vi "Test Lock-in amplifier API.vi"() -> ()   [LabVIEW 2020]
doc: "Lock-in amplifier API Tester."
uses:
  Lock-in amplifier.lvlib
  <vilib>/Utility/error.llb/DialogType.ctl
  Support/Filter config -- cluster.ctl
  Support/Input signal config -- typedef.ctl
  Support/Sense-Reserve config -- cluster.ctl
panel:
  in  "Sens/Reserve":T1={"Dynamic Reserve "=1, "Sensitivity"=20} {"Dynamic Reserve" items=["Auto Reserve"=-1, "High Reserve"=0, "Normal"=1, "Low Noise"=2]; "Sensitivity" items=["Auto Gain"=-1, "2 nV/fA"=0, "5 nV/fA"=1, "10 nV/fA"=2, "20 nV/fA"=3, "50 nV/fA"=4, "100 nV/fA"=5, "200 nV/fA"=6, "500 nV/fA"=7, "1 uV/pA"=8, "2 uV/pA"=9, "5 uV/pA"=10, "10 uV/pA"=11, "20 uV/pA"=12, "50 uV/pA"=13, "100 uV/pA"=14, "200 uV/pA"=15, "500 uV/pA"=16, "1 mV/nA"=17, "2 mV/nA"=18, "5 mV/nA"=19, "10 mV/nA"=20, "20 mV/nA"=21, "50 mV/nA"=22, "100 mV/nA"=23, "200 mV/nA"=24, "500 mV/mA"=25, "1 V/uA"=26]}
  in  "Input signal":T2={"Input Shield Grounding"=1, "Input Connection"=0, "Input Coupling"=1} {"Input Shield Grounding" items=["Float", "Ground"]; "Input Connection" items=["Single-Ended Voltage", "Differential Voltage", "1 MOhm Current Gain", "100 MOhm Current Gain"]; "Input Coupling" items=["AC", "DC"]}
  in  "Filter":T3={"Time Constant"=9, "Enable Sync Filter?"=FALSE, "Low Pass Filter Slope"=1} {"Low Pass Filter Slope" items=["6 dB/oct", "12 dB/oct", "18 db/oct", "24 dB/oct"]; "Time Constant" items=["10 us", "30 us", "100 us", "300 us", "1 ms", "3 ms", "10 ms", "30 ms", "100 ms", "300 ms", "1 s", "3 s", "10 s", "30 s", "100 s", "300 s", "1 ks", "3 ks", "10 ks", "30 ks"]}
  in  "Timeout":i32=100
  in  "Stop continuous acquisition":bool
  in  "Average?":bool
  in  "Start continuous acquisition":bool
  in  "Configure":bool
  out "Connected":bool
  in  "Simulate?":bool
  in  "Disconnect":bool
  in  "N samples":i32
  in  "Average samples":bool
  in  "Parameter":u16(ring)=1 items=["X"=1, "Y"=2, "R"=3, "Theta"=4, "Channel 1"=5, "Channel 2"=6, "Aux In 1"=7, "Aux In 2"=8, "Aux In 3"=9, "Aux In 4"=10]
  out "Data":dbl
  in  "Read datapoint":bool
  in  "VISA resource name":refnum<visa-resource-name>
  in  "Connect":bool
  in  "Remove Panel from Subpanel":bool
  in  "Draw Panel into Subpanel":bool
  in  "Show Diagram on Init":bool
  in  "Run as Singleton?":bool
  in  "Show Block Diagram":bool
  in  "Refresh Modules":bool
  out "Active Modules":string[](array[string])
  in  "Stop Module":bool
  in  "Select Module":i32(ring)=-1 caption="Select Module\nTo send Request to" items=["All"=-1]
  in  "Run New Module":bool
  in  "Hide Module Panel":bool
  in  "Show Module Panel":bool
  out "Status":string
  # "This VI tests the API for the Module."
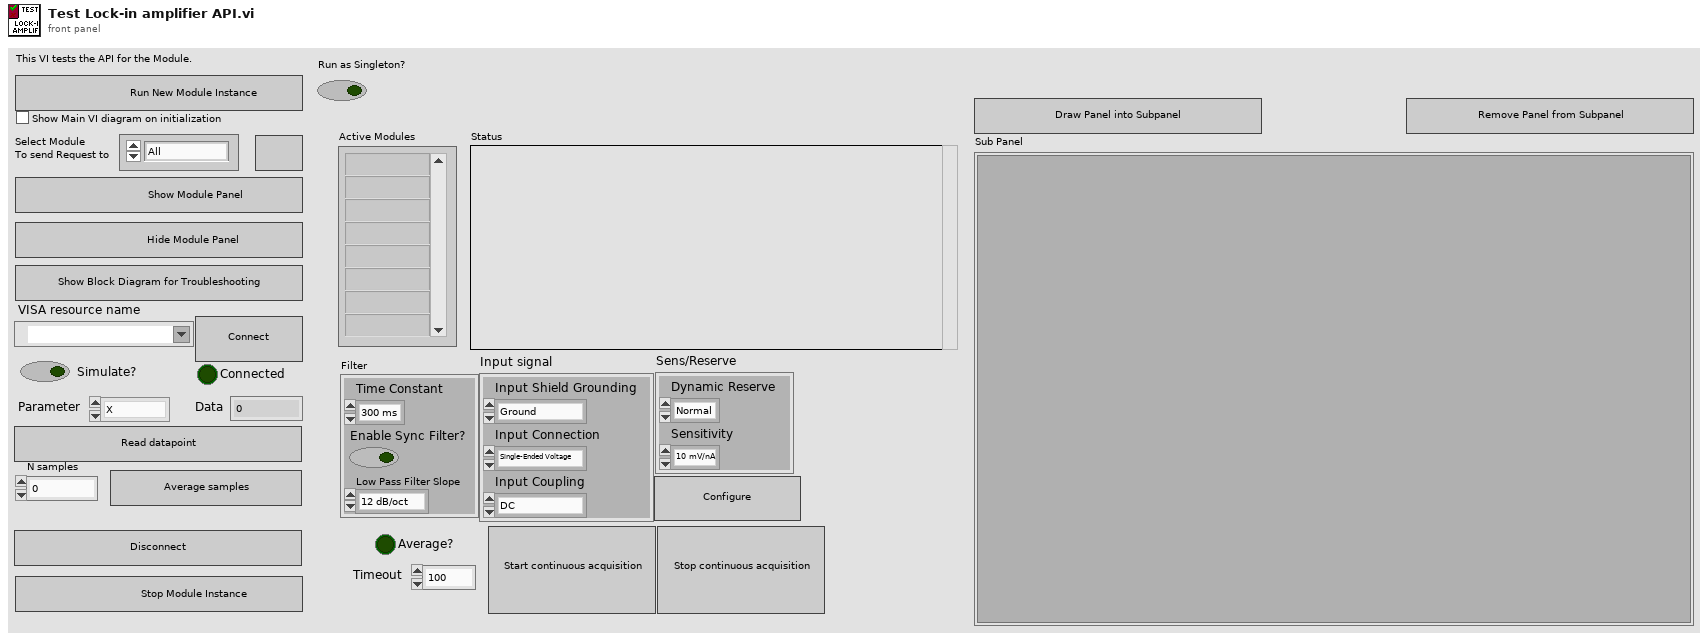
[diagram p1: front panel]
types:
  T1 = typedef "Lock-in amplifier.lvlib/Sense-Reserve config -- cluster.ctl" = cluster{"Dynamic Reserve ":i16, "Sensitivity":i16}
  T2 = typedef "Lock-in amplifier.lvlib/Input signal config -- typedef.ctl" = cluster{"Input Shield Grounding":u16, "Input Connection":u16, "Input Coupling":u16}
  T3 = typedef "Lock-in amplifier.lvlib/Filter config -- cluster.ctl" = cluster{"Time Constant":u16, "Enable Sync Filter?":bool, "Low Pass Filter Slope":u16}
  T4 = typedef "Lock-in amplifier.lvlib/Broadcast Events--cluster.ctl" = cluster{"Module Did Init":refnum<user-event>, "Status Updated":refnum<user-event>, "Error Reported":refnum<user-event>, "Module Did Stop":refnum<user-event>, "Update Module Execution Status":refnum<user-event>, "Helper Loop Status Updated":refnum<user-event>, "Data available":refnum<user-event>}
  T5 = typedef "DialogType.ctl" = u16
  T6 = typedef "Lock-in amplifier.lvlib/Helper Loop Status--enum.ctl" = enum16{"Awake", "Asleep"}
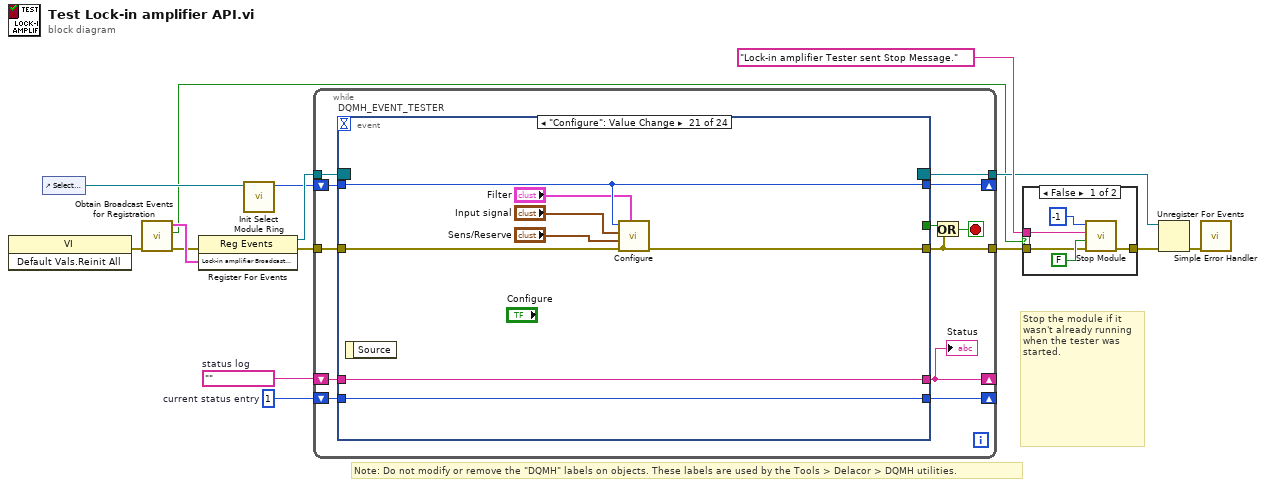
[diagram p0: block diagram]
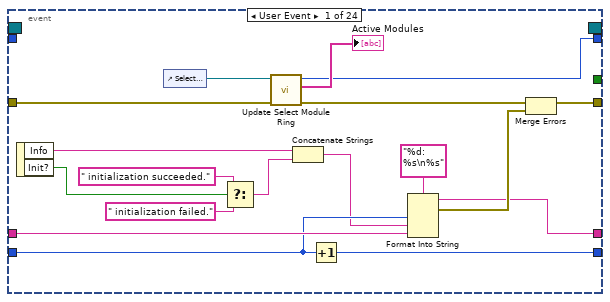
[diagram p3: hidden frame]
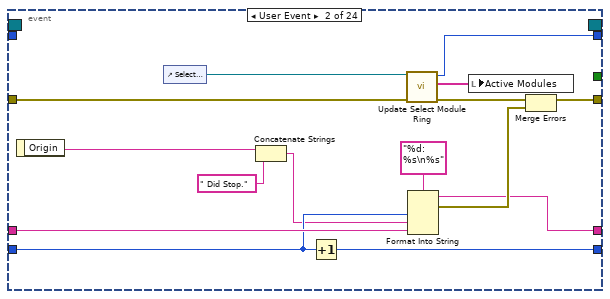
[diagram p4: hidden frame]
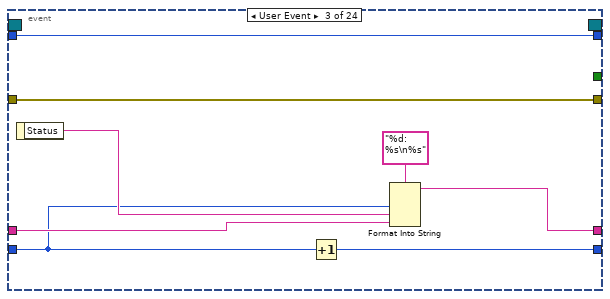
[diagram p5: hidden frame]
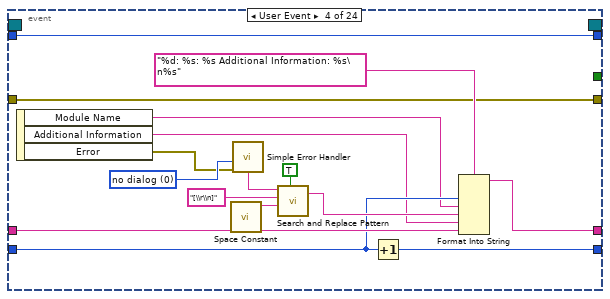
[diagram p6: hidden frame]
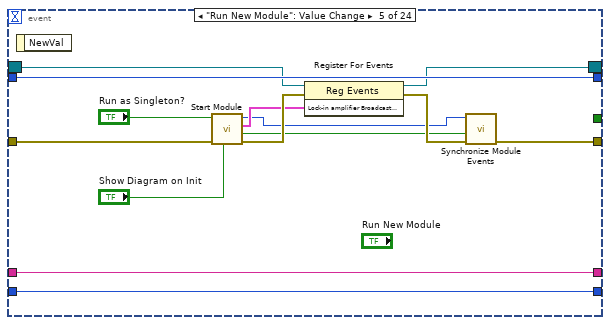
[diagram p7: hidden frame]
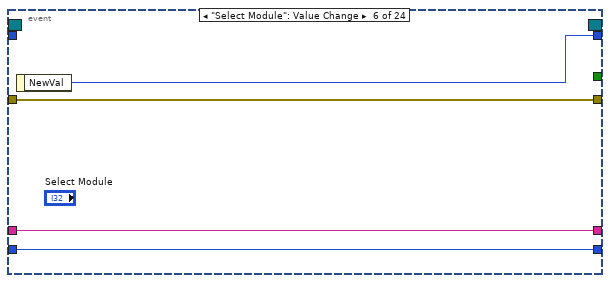
[diagram p8: hidden frame]
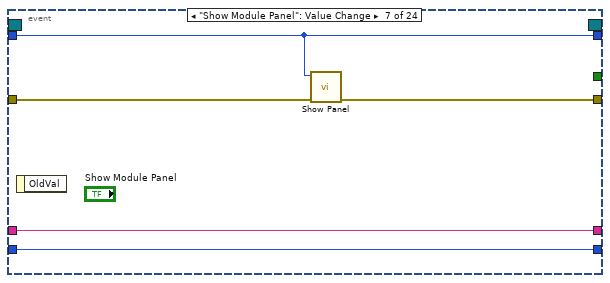
[diagram p9: hidden frame]
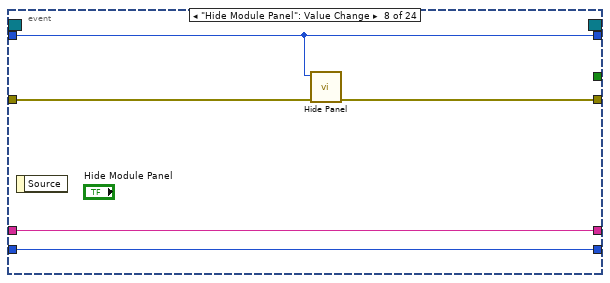
[diagram p10: hidden frame]
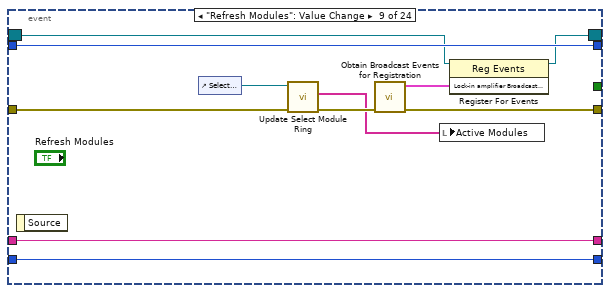
[diagram p11: hidden frame]
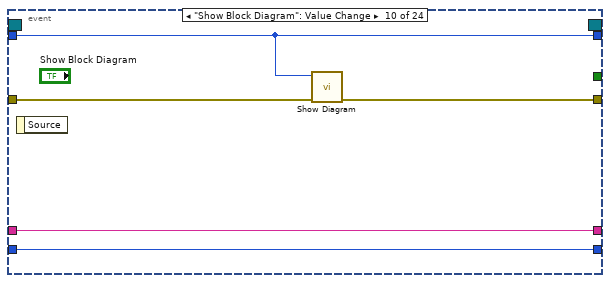
[diagram p12: hidden frame]
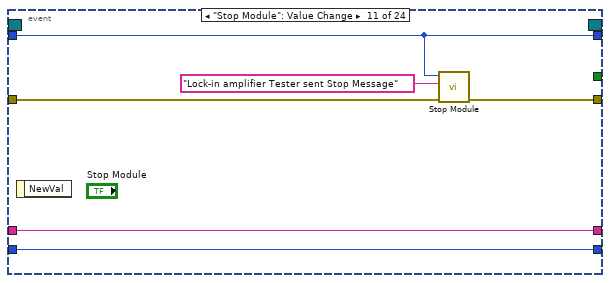
[diagram p13: hidden frame]
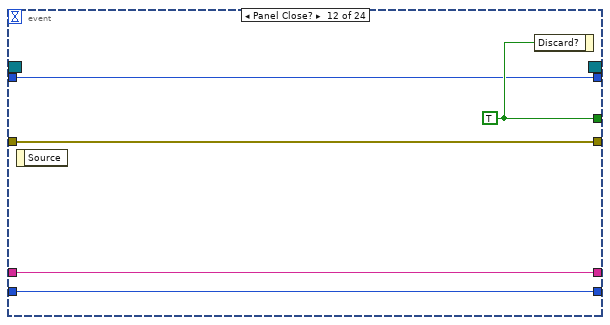
[diagram p14: hidden frame]
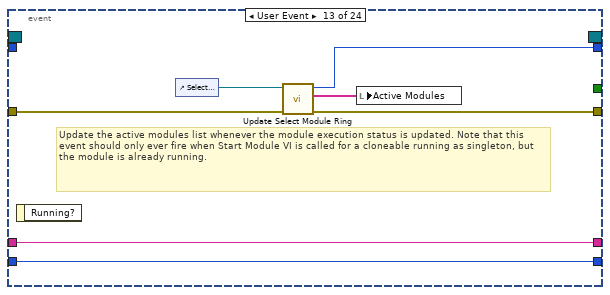
[diagram p15: hidden frame]
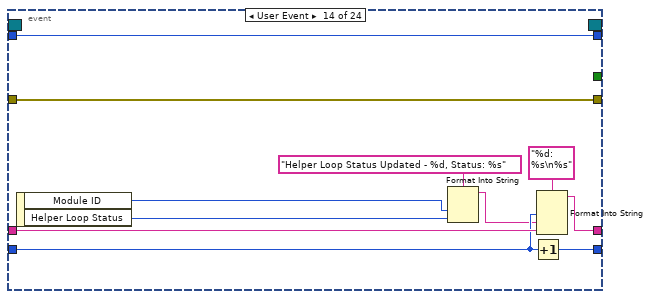
[diagram p16: hidden frame]
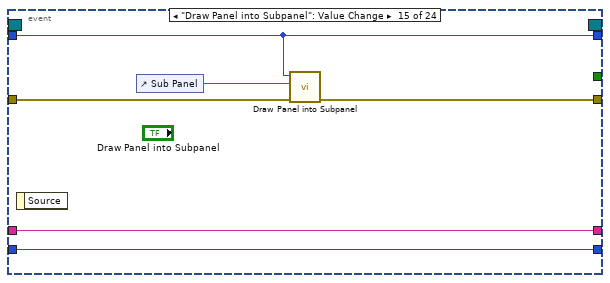
[diagram p17: hidden frame]
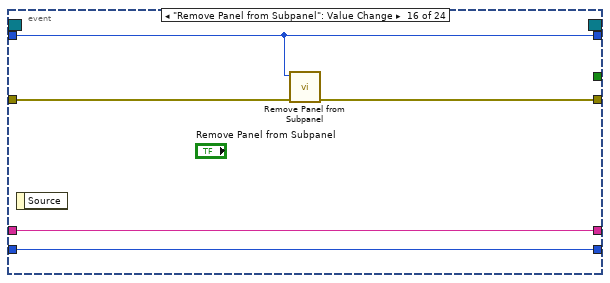
[diagram p18: hidden frame]
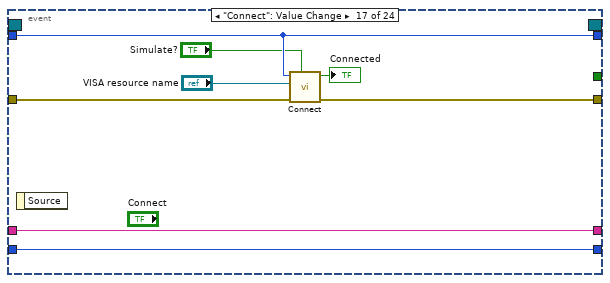
[diagram p19: hidden frame]
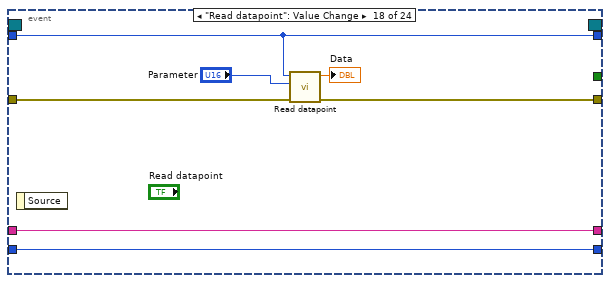
[diagram p20: hidden frame]
diagram:
  w12 = 1  # current status entry
  w13 = ""  # status log
  # "Stop the module if it wasn't already running when the tester was started."
  # "Note: Do not modify or remove the \"DQMH\" labels on objects. These labels are used by the Tools > Delacor > DQMH utilities."
  n1 = invoke class="VI" method="Default Vals.Reinit All"() -> (error out=w5:errorcluster)  [unwired: 3 in, 2 out]
  n2 = control-ref of="Select Module"() -> (w10:refnum<vi>)
  n3 = call "Obtain Broadcast Events for Registration.vi"("error in"=w5) -> ("error out"=w4:errorcluster, "Already running?"=w3:bool, "Lock-in amplifier Broadcast Events"=w9:T4)  [unwired: 8 in]
  n4 = register-events(error in=w4, w9) -> (reference out=w15:refnum<event-registration>, error out=w8:errorcluster)  [unwired: 1 in]
  n5 = call "Init Select Module Ring.vi"("Select Module Ring Ref"=w10) -> ("Value for All Modules"=w11:i32)  [unwired: 8 in, 2 out]
  n6 = while {
    tunnel: w15 -> [w27]
    tunnel: [w16] -> w2
    tunnel: w8 -> [w25]
    shift-right: [w21] -> _
    shift-left: w13 -> [w23]
    shift-right: [w22] -> _
    shift-left: w12 -> [w24]
    shift-right: [w18] -> _
    shift-left: w11 -> [w19]
    tunnel: [w17] -> w6
    stop <- w20 stop-if-true
    n7 = event "DQMH_EVENT_TESTER" shown="[20] \"Configure\": Value Change" {
      selector: w27 -> [_ _ _ _ w92 _ _ _ w118 _ _ _ _ _ _ _ _ _ _ _ _ _ _ _]
      dyn-events: [_ _ _ _ w91 _ _ _ w117 _ _ _ _ _ _ _ _ _ _ _ _ _ _ _] -> w17
      timeout: _ -> [_ _ _ _ _ _ _ _ _ _ _ _ _ _ _ _ _ _ _ _ _ _ _ _]
      tunnel: [_ _ _ _ _ _ _ _ _ _ _ w139 _ _ _ _ _ _ _ _ _ _ _ _] -> w26
      tunnel: [w35 w52 w68 w72 w90 w102 w106 w111 w114 w125 w130 w138 w142 w157 w160 w165 w173 w180 w188 w193 w201 w210 w215 w229] -> w16
      tunnel: w25 -> [w37 w54 w68 w72 w93 w102 w107 w112 w119 w128 w131 w138 w143 w157 w163 w168 w176 w183 w191 w196 w204 w213 w218 w229]
      tunnel: w24 -> [w42 w57 w61 w75 w95 w100 w104 w109 w122 w126 w133 w136 w145 w153 w161 w166 w174 w181 w189 w194 w202 w211 w216 w225]
      tunnel: w23 -> [w43 w58 w64 w76 w96 w101 w105 w110 w123 w127 w134 w137 w146 w155 w162 w167 w175 w182 w190 w195 w203 w212 w217 w227]
      tunnel: [w40 w55 w65 w74 w96 w101 w105 w110 w123 w127 w134 w137 w146 w154 w162 w167 w175 w182 w190 w195 w203 w212 w217 w226] -> w21
      tunnel: [w41 w56 w67 w73 w95 w100 w104 w109 w122 w126 w133 w136 w145 w152 w161 w166 w174 w181 w189 w194 w202 w211 w216 w224] -> w22
      tunnel: w19 -> [_ _ w62 w84 w94 _ w103 w108 w121 w124 w132 w135 _ w156 w159 w164 w172 w179 w187 w192 w200 w209 w214 w228]
      tunnel: [w32 w49 w62 w84 w94 w99 w103 w108 w121 w124 w132 w135 w141 w156 w159 w164 w172 w179 w187 w192 w200 w209 w214 w228] -> w18
      event User Event {
        n8 = event-data() -> ("Info"=w39:string, "Init?"=w29:bool)  [unwired: 1 in]
        n9 = control-ref of="Select Module"() -> (w34:refnum<vi>)
        n10 = Select(t=" initialization succeeded.", s=w29, f=" initialization failed.") -> (s? t:f=w28:string)
        n11 = call "Update Select Module Ring.vi"("error in (no error)"=w37, "Select Module Ring Ref"=w34) -> ("error out"=w36:errorcluster, "Active Modules (Array)"=→"Active Modules":string[], "New Module Ring Value"=w32:i32)  [unwired: 7 in]
        n12 = Concatenate Strings(w39, w28) -> (w38:string)
        n13 = Increment(x=w42) -> (x+1=w41:i32)
        n14 = Format Into String(format string="%d: %s\n%s", w42, w38, w43) -> (resulting string=w40:string, error out=w45:errorcluster)  [unwired: 2 in]
        n15 = Merge Errors(w36, w45) -> (w35:errorcluster)
      }
      event User Event {
        n16 = event-data() -> ("Origin"=w47:string)  [unwired: 1 in]
        n17 = control-ref of="Select Module"() -> (w51:refnum<vi>)
        n18 = Concatenate Strings(w47, " Did Stop.") -> (w46:string)
        n19 = Increment(x=w57) -> (x+1=w56:i32)
        n20 = call "Update Select Module Ring.vi"("error in (no error)"=w54, "Select Module Ring Ref"=w51) -> ("error out"=w53:errorcluster, "Active Modules (Array)"=w50:string[], "New Module Ring Value"=w49:i32)  [unwired: 7 in]
        n21 = Format Into String(format string="%d: %s\n%s", w57, w46, w58) -> (resulting string=w55:string, error out=w60:errorcluster)  [unwired: 2 in]
        n22 = local write "Active Modules"(w50) -> ()
        n23 = Merge Errors(w53, w60) -> (w52:errorcluster)
      }
      event User Event {
        n24 = event-data() -> ("Status"=w63:string)  [unwired: 1 in]
        n25 = Increment(x=w61) -> (x+1=w67:i32)
        n26 = Format Into String(format string="%d: %s\n%s", w61, w63, w64) -> (resulting string=w65:string)  [unwired: 2 in, 1 out]
      }
      event User Event {
        w77 = T5 0 items=["no dialog", "OK message", "continue or stop message", "OK message + warnings", "continue/stop + warnings"] ("type of dialog (OK msg:1)")
        n27 = event-data() -> ("Module Name"=w71:string, "Additional Information"=w70:string, "Error"=w69:errorcluster)  [unwired: 1 in]
        n28 = call <vilib>:"Space Constant.vi"() -> ("String"=w81:string)
        n29 = call <vilib>:"Simple Error Handler.vi"("type of dialog (OK msg:1)"=w77, "error in (no error)"=w69) -> ("message"=w78:string)  [unwired: 3 in, 4 out]
        n30 = call <vilib>:"Search and Replace Pattern.vi"("string"=w78, "regular expression (\"\")"="[\\r\\n]" ("regular expression (\"\")"), "replace string (\"\")"=w81, "replace all? (F)"=TRUE ("replace all CR/LF with spaces")) -> ("result string"=w79:string)  [unwired: 1 in, 1 out]
        n31 = Increment(x=w75) -> (x+1=w73:i32)
        n32 = Format Into String(format string="%d: %s: %s Additional Information: %s\n%s", w75, w71, w79, w70, w76) -> (resulting string=w74:string)  [unwired: 2 in, 1 out]
      }
      event "Run New Module": Value Change {
        n33 = event-data() -> ()  [unwired: 1 in, 1 out]
        n34 = call "Start Module.vi"("Show Main VI Diagram on Init (F)"="Show Diagram on Init", "error in"=w93, "Run as Singleton? (F)"="Run as Singleton?") -> ("error out"=w97:errorcluster, "Wait for Event Sync?"=w89:bool, "Lock-in amplifier Broadcast Events"=w88:T4, "Module ID"=w85:i32)  [unwired: 5 in]
        n35 = register-events(reference=w92, error in=w97, w88) -> (reference out=w91:refnum<event-registration>, error out=w98:errorcluster)
        n36 = call "Synchronize Module Events.vi"("error in"=w98, "Wait for Event Sync?"=w89, "Module ID in"=w85) -> ("error out"=w90:errorcluster)  [unwired: 7 in, 1 out]
      }
      event "Select Module": Value Change {
        n37 = event-data() -> ("NewVal"=w99:i32)  [unwired: 1 in]
      }
      event "Show Module Panel": Value Change {
        n38 = event-data() -> ()  [unwired: 1 in, 1 out]
        n39 = call "Show Panel.vi"("error in (no error)"=w107, "Module ID"=w103) -> ("error out"=w106:errorcluster)  [unwired: 9 in]
      }
      event "Hide Module Panel": Value Change {
        n40 = event-data() -> ()  [unwired: 1 in, 1 out]
        n41 = call "Hide Panel.vi"("error in (no error)"=w112, "Module ID"=w108) -> ("error out"=w111:errorcluster)  [unwired: 9 in]
      }
      event "Refresh Modules": Value Change {
        n42 = event-data() -> ()  [unwired: 1 in, 1 out]
        n43 = control-ref of="Select Module"() -> (w120:refnum<vi>)
        n44 = call "Update Select Module Ring.vi"("error in (no error)"=w119, "Select Module Ring Ref"=w120) -> ("error out"=w115:errorcluster, "Active Modules (Array)"=w113:string[])  [unwired: 7 in, 1 out]
        n45 = call "Obtain Broadcast Events for Registration.vi"("error in"=w115) -> ("error out"=w114:errorcluster, "Lock-in amplifier Broadcast Events"=w116:T4)  [unwired: 8 in, 1 out]
        n46 = local write "Active Modules"(w113) -> ()
        n47 = register-events(reference=w118, w116) -> (reference out=w117:refnum<event-registration>)  [unwired: 1 in, 1 out]
      }
      event "Show Block Diagram": Value Change {
        n48 = event-data() -> ()  [unwired: 1 in, 1 out]
        n49 = call "Show Diagram.vi"("error in (no error)"=w128, "Module ID"=w124) -> ("error out"=w125:errorcluster)  [unwired: 9 in]
      }
      event "Stop Module": Value Change {
        n50 = event-data() -> ()  [unwired: 1 in, 1 out]
        n51 = call "Stop Module.vi"("error in"=w131, "Origin"="Lock-in amplifier Tester sent Stop Message", "Module ID"=w132) -> ("error out"=w130:errorcluster)  [unwired: 8 in]
      }
      event Panel Close? {
        w139 = TRUE ("Discard?")
        n52 = event-data() -> ()  [unwired: 1 in, 1 out]
        n53 = event-data("Discard?"=w139) -> ()  [unwired: 1 in, 1 out]
      }
      event User Event {
        # "Update the active modules list whenever the module execution status is updated. Note that this event should only ever fire when Start Module VI is called for a cloneable running as singleton, but the module is already running."
        n54 = event-data() -> ()  [unwired: 1 in, 1 out]
        n55 = control-ref of="Select Module"() -> (w144:refnum<vi>)
        n56 = call "Update Select Module Ring.vi"("error in (no error)"=w143, "Select Module Ring Ref"=w144) -> ("error out"=w142:errorcluster, "Active Modules (Array)"=w140:string[], "New Module Ring Value"=w141:i32)  [unwired: 7 in]
        n57 = local write "Active Modules"(w140) -> ()
      }
      event User Event {
        n58 = event-data() -> ("Module ID"=w148:i32, "Helper Loop Status"=w147:T6)  [unwired: 1 in]
        n59 = Format Into String(format string="Helper Loop Status Updated - %d, Status: %s", w148, w147) -> (resulting string=w149:string)  [unwired: 2 in, 1 out]
        n60 = Increment(x=w153) -> (x+1=w152:i32)
        n61 = Format Into String(format string="%d: %s\n%s", w153, w149, w155) -> (resulting string=w154:string)  [unwired: 2 in, 1 out]
      }
      event "Draw Panel into Subpanel": Value Change {
        n62 = event-data() -> ()  [unwired: 1 in, 1 out]
        n63 = control-ref of="Sub Panel"() -> (w158:refnum<vi>)
        n64 = call "Draw Panel into Subpanel.vi"("error in"=w163, "Sub Panel"=w158, "Module ID"=w159) -> ("error out"=w160:errorcluster)  [unwired: 8 in]
      }
      event "Remove Panel from Subpanel": Value Change {
        n65 = event-data() -> ()  [unwired: 1 in, 1 out]
        n66 = call "Remove Panel from Subpanel.vi"("error in"=w168, "Module ID"=w164) -> ("error out"=w165:errorcluster)  [unwired: 9 in]
      }
      event "Connect": Value Change {
        n67 = event-data() -> ()  [unwired: 1 in, 1 out]
        n68 = call "Connect.vi"("Simulate?"="Simulate?", "error in"=w176, "VISA resource name"="VISA resource name", "Module ID"=w172) -> ("error out"=w173:errorcluster, "Connection successful?"=→"Connected":bool)  [unwired: 5 in, 1 out]
      }
      event "Read datapoint": Value Change {
        n69 = event-data() -> ()  [unwired: 1 in, 1 out]
        n70 = call "Read datapoint.vi"("error in"=w183, "Parameter"="Parameter", "Module ID"=w179) -> ("error out"=w180:errorcluster, "Data"=→"Data":dbl)  [unwired: 6 in, 1 out]
      }
      event "Average samples": Value Change {
        n71 = event-data() -> ()  [unwired: 1 in, 1 out]
        n72 = local read "Parameter"() -> (w185:u16)
        n73 = call "Average samples.vi"("error in"=w191, "N samples"="N samples", "Parameter"=w185, "Module ID"=w187) -> ("error out"=w188:errorcluster, "Measurement"=w184:dbl)  [unwired: 5 in, 1 out]
        n74 = local write "Data"(w184) -> ()
      }
      event "Disconnect": Value Change {
        n75 = event-data() -> ()  [unwired: 1 in, 1 out]
        n76 = call "Disconnect.vi"("error in"=w196, "Module ID"=w192) -> ("error out"=w193:errorcluster)  [unwired: 9 in]
      }
      event "Configure": Value Change {
        n77 = event-data() -> ()  [unwired: 1 in, 1 out]
        n78 = call "Configure.vi"("Filter"="Filter", "error in"=w204, "Sens/Reserve"="Sens/Reserve", "Input signal"="Input signal", "Module ID"=w200) -> ("error out"=w201:errorcluster)  [unwired: 6 in]
      }
      event "Start continuous acquisition": Value Change {
        n79 = event-data() -> ()  [unwired: 1 in, 1 out]
        n80 = local read "N samples"() -> (w206:i32)
        n81 = local read "Parameter"() -> (w208:u16)
        n82 = call "Start continuous acquisition.vi"("N-samples"=w206, "Timeout"="Timeout", "Average?"="Average?", "error in"=w213, "Parameter"=w208, "Module ID"=w209) -> ("error out"=w210:errorcluster)  [unwired: 5 in]
      }
      event "Stop continuous acquisition": Value Change {
        n83 = event-data() -> ()  [unwired: 1 in, 1 out]
        n84 = call "Stop continuous acquisition.vi"("error in"=w218, "Module ID"=w214) -> ("error out"=w215:errorcluster)  [unwired: 9 in]
      }
      event User Event {
        n85 = event-data() -> ("Data"=w219:dbl)  [unwired: 1 in]
        n86 = local write "Data"(w219) -> ()
        n87 = Format Into String(format string="Response Received - %s %0.6f", "Data ready: " ("input 1"), w219) -> (resulting string=w221:string)  [unwired: 2 in, 1 out]
        n88 = Increment(x=w225) -> (x+1=w224:i32)
        n89 = Format Into String(format string="%d: %s\n%s", w225, w221, w227) -> (resulting string=w226:string)  [unwired: 2 in, 1 out]
      }
    }
    "Status" <- w21
    n90 = Or(x=w26, y=w16) -> (x .or. y?=w20:bool)
  }
  n91 = case shown="False" w3 {
    tunnel: [w234 w235] -> w14
    tunnel: "Lock-in amplifier Tester sent Stop Message." ("Origin") -> [w233 _]
    tunnel: w2 -> [w230 w235]
    frame False {
      n92 = call "Stop Module.vi"("error in"=w230, "Wait for Module to stop? (F)"=FALSE ("Wait for Module to stop?"), "Origin"=w233, "Module ID"=-1 ("Stop all")) -> ("error out"=w234:errorcluster)  [unwired: 7 in]
    }
    frame True {
    }
  }
  n93 = Unregister For Events(event registration refnum=w6, error in=w14) -> (error out=w1:errorcluster)
  n94 = call <vilib>:"Simple Error Handler.vi"("error in (no error)"=w1) -> ()  [unwired: 4 in, 5 out]
